vi "tm_closecamera.vi"(8 "error in (no error)":errorcluster {"code" format="%.0x"}, 11 "Handle in":u32) -> (0 "error out":errorcluster {"code" format="%.0x"})   [LabVIEW 2023]
uses:
  tmcamcon.dll
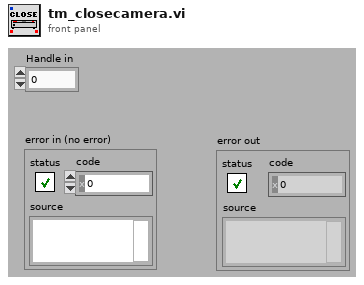
[diagram p1: front panel]
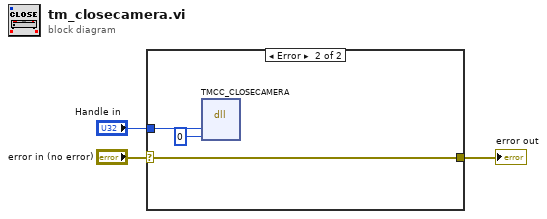
[diagram p0: block diagram]
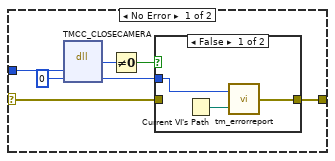
[diagram p2: hidden frame]
diagram:
  n1 = case shown="Error" "error in (no error)" {
    selector: "error in (no error)" -> [w7 w15]
    tunnel: [w6 w15] -> w2
    tunnel: "Handle in" -> [w8 w16]
    frame No Error {
      n2 = dll-call lib="tmcamcon.dll" fn="TMCC_CLOSECAMERA"("index"=w8, "Erval"=0) -> ("return type"=w10:u32, "Erval"=w5:i32)  [unwired: 4 in, 2 out]
      n3 = Not Equal To 0?(x=w10) -> (x != 0?=w4:bool)
      n4 = case shown="False" w4 {
        tunnel: w7 -> [_ w14]
        tunnel: [w12 w14] -> w6
        tunnel: w5 -> [w11 _]
        frame False {
          n5 = Current VI's Path() -> (path=w13:path)
          n6 = call "tm_errorreport.vi"("Source"=w13, "Error"=w11) -> ("error out"=w12:errorcluster)
        }
        frame True {
        }
      }
    }
    frame Error {
      n7 = dll-call lib="tmcamcon.dll" fn="TMCC_CLOSECAMERA"("HDCAM"=w16, "Erval"=0) -> ()  [unwired: 6 in, 2 out]
    }
  }
  "error out" <- w2
